vi "Problem 1 - Multiples of 3 and 5.vi"() -> ()   [LabVIEW 2021, in "Project Euler.lvlib"]
uses:
  Project Euler.lvlib
  Utilities/Numeric Utilities/Numeric Utilities.lvlib
panel:
  out "No. of elements of array A":i32
  out "sum of array A":i32
  out "Natural numbers that are divisible by 3 or by 5 (array A)":i32[](array[numeric])
  out "x":i32
  # "Development\nControls or indicators that are useful for development or testing, but which are not outputs of the VI."
  # "Input\nInputs to the VI"
  # "Output\nOutputs of the VI"
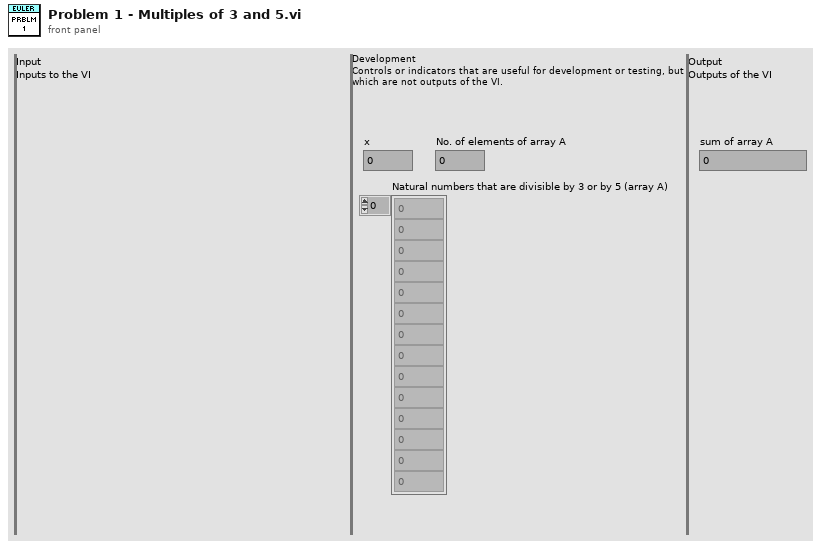
[diagram p1: front panel]
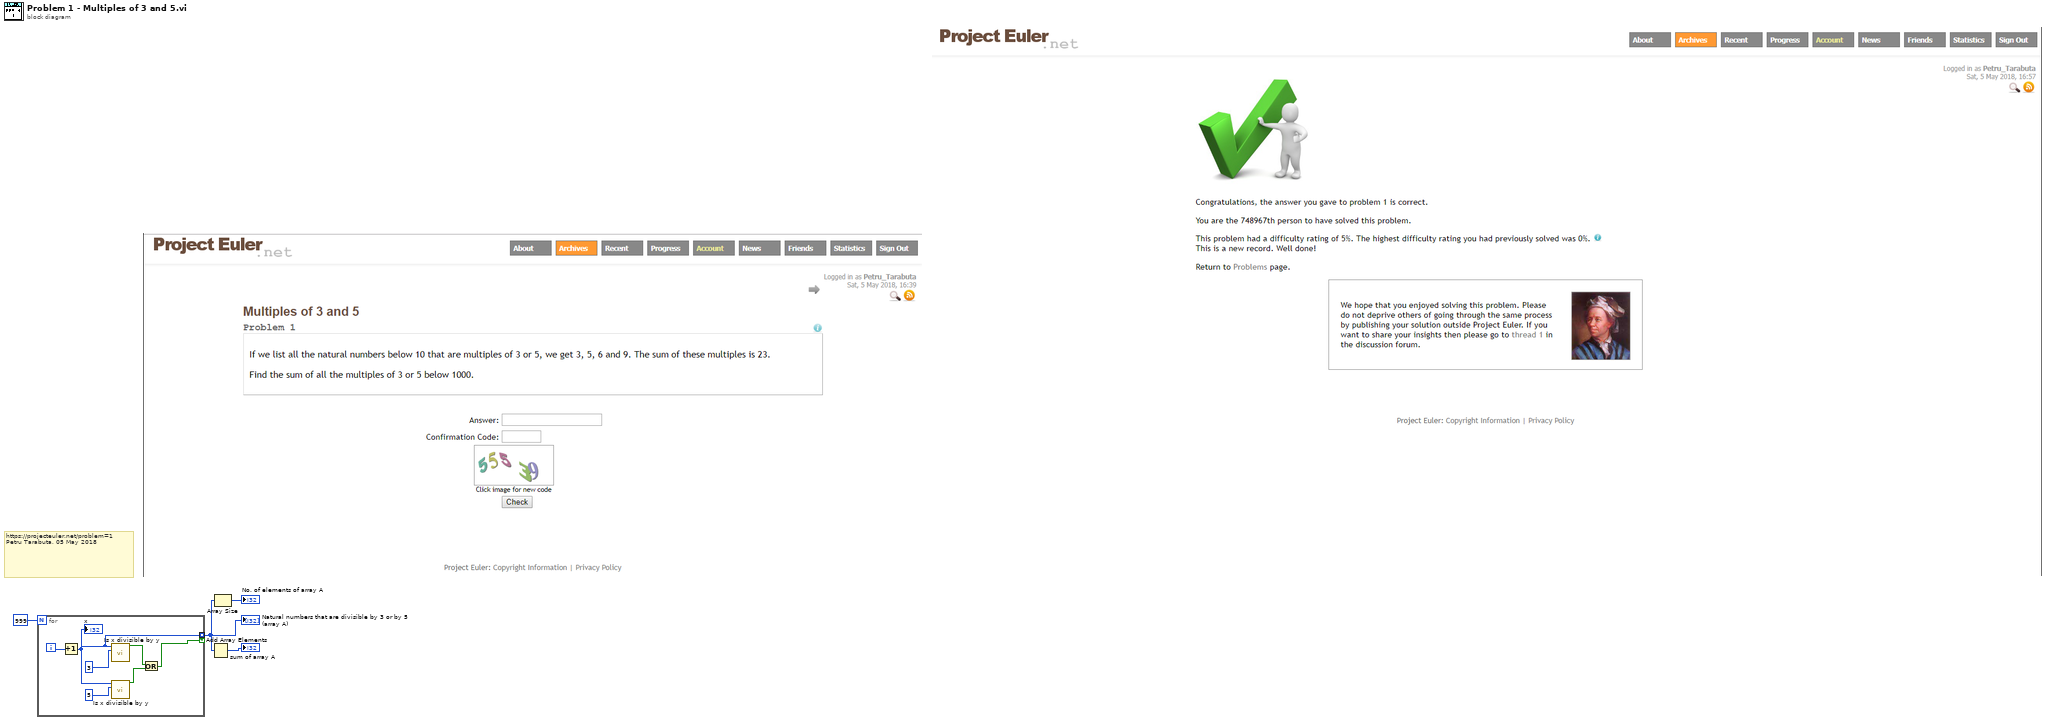
[diagram p0: block diagram]
diagram:
  # "https://projecteuler.net/problem=1\nPetru Tarabuta, 05 May 2018"
  n1 = for {
    N: 999 -> [_]
    tunnel: [w6] -> w2 mode=indexing if=w5
    i -> [w11]
    n2 = Increment(x=w11) -> (x+1=w6:i32)
    "x" <- w6
    n3 = call "Is x divisible by y.vi"("y"=3, "x"=w6) -> ("T = x is divisible by y"=w9:bool)  [unwired: 7 in, 2 out]
    n4 = call "Is x divisible by y.vi"("y"=5, "x"=w6) -> ("T = x is divisible by y"=w7:bool)  [unwired: 7 in, 2 out]
    n5 = Or(x=w9, y=w7) -> (x .or. y?=w5:bool)
  }
  "Natural numbers that are divisible by 3 or by 5 (array A)" <- w2
  n6 = Add Array Elements(numeric array=w2) -> (sum=→"sum of array A":i32)
  n7 = Array Size(array=w2) -> (size(s)=→"No. of elements of array A":i32)
